vi "Convex Hull 3D (GiftWrap).vi"(0 "Vertices":sgl[][](array[numeric])=[[0.0, 0.0, 0.0], [1.0, 0.0, 0.0], [1.0, 1.0, 0.0], [0.0, 1.0, 0.0], [0.0, 0.0, 1.0], [1.0, 0.0, 1.0], [1.0, 1.0, 1.0], [0.0, 1.0, 1.0], [10.0, 10.0, 0.0], [11.0, 10.0, 0.0], [11.0, 11.0, 0.0], [10.0, 11.0, 0.0], [10.0, 10.0, 1.0], [11.0, 10.0, 1.0], [11.0, 11.0, 1.0], [10.0, 11.0, 1.0]]) -> (1 "Convex hull triangles (partial proc.)":T1[](array[typedef]), 2 "Stack error":errorcluster)   [LabVIEW 2014]
uses:
  Typedefs/Triangle.ctl
  Typedefs/Edge.ctl
  Subroutines/Cross product 3D.vi
  Subroutines/Unit vector.vi
panel:
  # "PN 21/03/2015"
  # "Vertices"
  # "Edges"
  # "Unit normal"
  # "Edge unit normals"
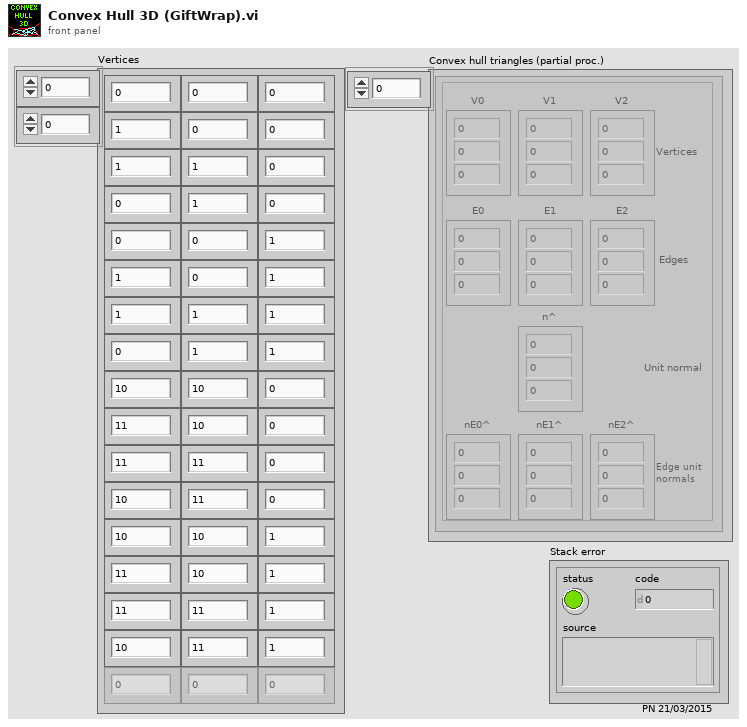
[diagram p1: front panel]
types:
  T1 = typedef "Triangle.ctl" = cluster{"V0":sgl[], "V1":sgl[], "V2":sgl[], "E0":sgl[], "E1":sgl[], "E2":sgl[], "n^":sgl[], "nE0^":sgl[], "nE1^":sgl[], "nE2^":sgl[]}
  T2 = typedef "Edge.ctl" = cluster{"V0":sgl[], "V1":sgl[], "E01":sgl[]}
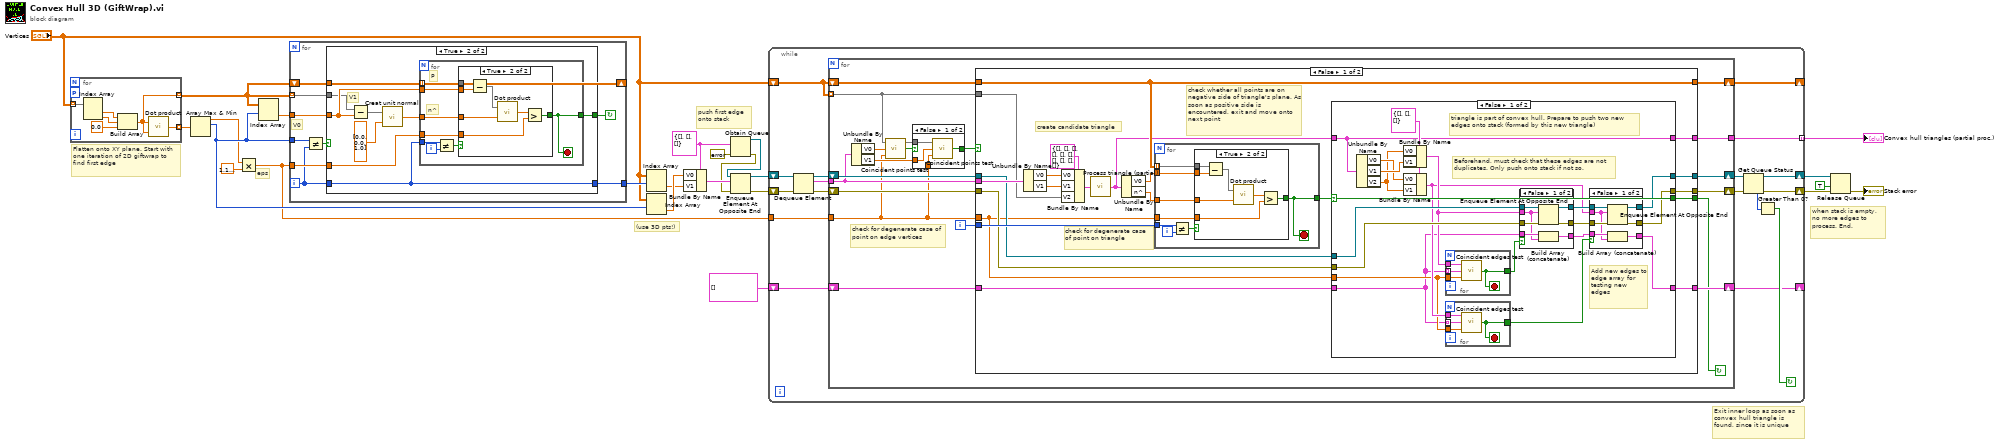
[diagram p0: block diagram]
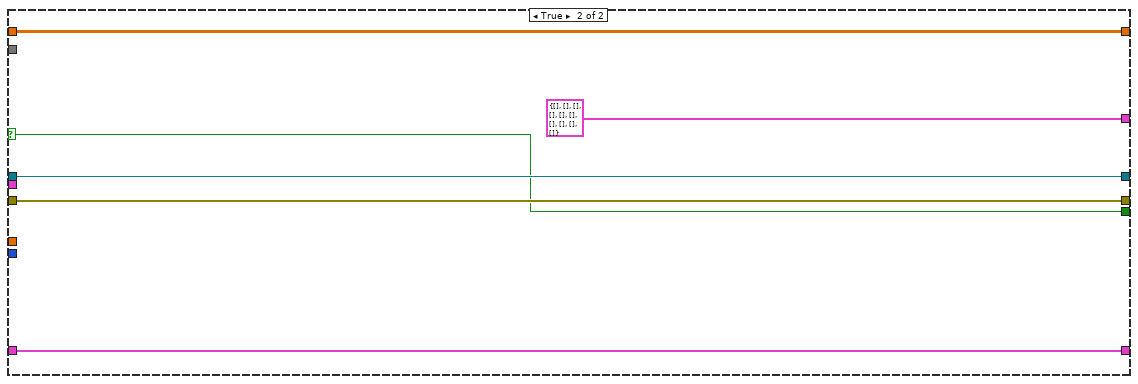
[diagram p7: hidden frame]
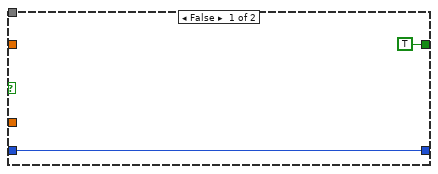
[diagram p8: hidden frame]
diagram:
  w12 = T2 {"V0"=[], "V1"=[], "E01"=[]} ("Edge")
  # "when stack is empty, no more edges to process. End."
  # "Exit inner loop as soon as convex hull triangle is found, since it is unique"
  # "(use 3D pts!)"
  # "push first edge onto stack"
  # "eps"
  # "Flatten onto XY plane. Start with one iteration of 2D giftwrap to find first edge"
  n1 = for {
    tunnel: "Vertices" -> [w30] mode=indexing
    tunnel: [w29] -> w24 mode=indexing
    workers-P: _ -> [_]
    tunnel: [w26] -> w22 mode=indexing
    n2 = Index Array(array=w30) -> (element #1=w28:sgl, element #2=w27:sgl)  [unwired: 2 in]
    n3 = Build Array(w28, w27, sgl 0.0 ("element")) -> (w26:sgl[])
    n4 = call "Dot product.vi"("B"=w26, "A"=w26) -> ("A . B"=w29:sgl)
  }
  n5 = Array Max & Min(array=w24) -> (max value=w4:sgl, max index (indices)=w13:i32)  [unwired: 2 out]
  n6 = Multiply(x=w4, y=sgl 1.1920929e-07) -> (x*y=w5:sgl)
  n7 = Index Array(array=w22, index (row)=w13) -> (element=w23:sgl[])  [unwired: 1 in]
  n8 = for {
    tunnel: w23 -> [w39]
    tunnel: w22 -> [w36] mode=indexing
    shift-right: [w37] -> _
    shift-left: w22 -> [w37]
    tunnel: w5 -> [w38]
    tunnel: [w33] -> w21
    tunnel: w13 -> [w31]
    i -> [w32]
    stop <- w35 continue-if-true
    # "V0"
    n9 = Not Equal?(x=w31, y=w32) -> (x != y?=w34:bool)
    n10 = case shown="True" w34 {
      tunnel: w39 -> [_ w48]
      tunnel: w38 -> [_ w47]
      tunnel: w37 -> [_ w46]
      tunnel: w36 -> [_ w45]
      tunnel: [TRUE w44] -> w35
      tunnel: w32 -> [w40 w42]
      tunnel: [w40 w42] -> w33
      frame False {
      }
      frame True {
        # "V1"
        n11 = Subtract(x=w45, y=w48) -> (x-y=w43:sgl[])
        n12 = call "Creat unit normal.vi"("E2"=sgl[] [0.0, 0.0, 1.0], "E1"=w43) -> ("n^ = (E1 x E2) / ||E1 x E2||"=w49:sgl[])
        n13 = for {
          tunnel: w49 -> [w55]
          tunnel: w46 -> [w54] mode=indexing
          tunnel: w42 -> [w57]
          tunnel: w48 -> [w53]
          tunnel: w47 -> [w52]
          tunnel: [w51] -> w44
          i -> [w58]
          stop <- w51 stop-if-true
          # "n^"
          # "P"
          n14 = Not Equal?(x=w57, y=w58) -> (x != y?=w56:bool)
          n15 = case shown="True" w56 {
            selector: w56 -> [w59 _]
            tunnel: w55 -> [_ w65]
            tunnel: w54 -> [_ w64]
            tunnel: w53 -> [_ w63]
            tunnel: w52 -> [_ w61]
            tunnel: [w59 w60] -> w51
            frame False {
            }
            frame True {
              n16 = Subtract(x=w64, y=w63) -> (x-y=w66:sgl[])
              n17 = call "Dot product.vi"("B"=w65, "A"=w66) -> ("A . B"=w62:sgl)
              n18 = Greater?(x=w62, y=w61) -> (0:w60:bool)
            }
          }
        }
      }
    }
  }
  n19 = Index Array(array="Vertices", index (row)=w21) -> (element=w10:sgl[])  [unwired: 1 in]
  n20 = Index Array(array="Vertices", index (row)=w13) -> (element=w11:sgl[])  [unwired: 1 in]
  n21 = Bundle By Name(cluster=w12, "V0"=w11, "V1"=w10) -> (w18:T2)
  n22 = Obtain Queue(element data type=w12, error in (no error)=errorcluster {"status"=FALSE, "code"=0, "source"=""}) -> (queue out=w19:refnum<queue>, error out=w16:errorcluster)  [unwired: 3 in, 1 out]
  n23 = Enqueue Element At Opposite End(queue=w19, element=w18, error in (no error)=w16) -> (queue out=w8:refnum<queue>, error out=w9:errorcluster)  [unwired: 1 in, 1 out]
  n24 = while {
    shift-right: [w78] -> _
    shift-left: "Vertices" -> [w80]
    shift-right: [w74] -> w15
    shift-left: w8 -> [w83]
    shift-right: [w72] -> w14
    shift-left: w9 -> [w82]
    tunnel: w5 -> [w79]
    tunnel: [w69] -> w3 mode=indexing
    shift-right: [w67] -> _
    shift-left: T2[] [] -> [w68]
    stop <- w70 continue-if-true
    n25 = Dequeue Element(queue=w83, error in (no error)=w82) -> (queue out=w77:refnum<queue>, element=w81:T2, error out=w76:errorcluster)  [unwired: 1 in, 1 out]
    n26 = for {
      tunnel: w80 -> [w89] mode=indexing
      tunnel: w81 -> [w93]
      shift-right: [w99] -> w78
      shift-left: w80 -> [w101]
      tunnel: w79 -> [w87]
      shift-right: [w95] -> w75
      shift-left: w77 -> [w97]
      shift-right: [w94] -> w73
      shift-left: w76 -> [w96]
      tunnel: [w98] -> w69
      shift-right: [w85] -> w67
      shift-left: w68 -> [w86]
      i -> [w100]
      stop <- w84 continue-if-true
      # "check for degenerate case of point on edge vertices"
      n27 = Unbundle By Name(w93) -> ("V0"=w92:sgl[], "V1"=w88:sgl[])
      n28 = call "Coincident points test.vi"("epsilon"=w87, "Point 2"=w92, "Point 1"=w89) -> ("Points are coincident"=w91:bool)
      n29 = case shown="False" w91 {
        selector: w91 -> [_ w106]
        tunnel: [w103 w106] -> w90
        tunnel: w89 -> [w105 _]
        tunnel: w88 -> [w104 _]
        tunnel: w87 -> [w102 _]
        frame False {
          n30 = call "Coincident points test.vi"("epsilon"=w102, "Point 2"=w104, "Point 1"=w105) -> ("Points are coincident"=w103:bool)
        }
        frame True {
        }
      }
      n31 = case shown="False" w90 {
        selector: w90 -> [_ w199]
        tunnel: w93 -> [w116 _]
        tunnel: w89 -> [w107 _]
        tunnel: w101 -> [w121 w202]
        tunnel: w87 -> [w109 _]
        tunnel: w100 -> [w118 _]
        tunnel: [w121 w202] -> w99
        tunnel: [w119 w199] -> w84
        tunnel: [w111 T1 {"V0"=[], "V1"=[], "V2"=[], "E0"=[], "E1"=[], "E2"=[], "n^"=[], "nE0^"=[], "nE1^"=[], "nE2^"=[]} ("Triangle out")] -> w98
        tunnel: w97 -> [w115 w201]
        tunnel: w96 -> [w117 w200]
        tunnel: [w114 w201] -> w95
        tunnel: [w113 w200] -> w94
        tunnel: w86 -> [w110 w198]
        tunnel: [w108 w198] -> w85
        frame False {
          # "check for degenerate case of point on triangle"
          # "check whether all points are on negative side of triangle's plane. As soon as positive side is encountered, exit and move onto next point"
          # "create candidate triangle"
          n32 = Unbundle By Name(w116) -> ("V0"=w126:sgl[], "V1"=w125:sgl[])
          n33 = Bundle By Name(cluster=T1 {"V0"=[], "V1"=[], "V2"=[], "E0"=[], "E1"=[], "E2"=[], "n^"=[], "nE0^"=[], "nE1^"=[], "nE2^"=[]} ("Triangle"), "V0"=w126, "V1"=w125, "V2"=w107) -> (w124:T1)
          n34 = call "Process triangle (partial).vi"("Triangle in"=w124) -> ("Triangle out"=w112:T1)
          n35 = Unbundle By Name(w112) -> ("V0"=w122:sgl[], "n^"=w123:sgl[])
          n36 = for {
            tunnel: w123 -> [w185]
            tunnel: w121 -> [w184] mode=indexing
            tunnel: w118 -> [w187]
            tunnel: w122 -> [w183]
            tunnel: w109 -> [w182]
            tunnel: [w181] -> w120
            i -> [w188]
            stop <- w181 stop-if-true
            n37 = Not Equal?(x=w187, y=w188) -> (x != y?=w186:bool)
            n38 = case shown="True" w186 {
              selector: w186 -> [w189 _]
              tunnel: w185 -> [_ w195]
              tunnel: w184 -> [_ w194]
              tunnel: w183 -> [_ w193]
              tunnel: w182 -> [_ w191]
              tunnel: [w189 w190] -> w181
              frame False {
              }
              frame True {
                n39 = Subtract(x=w194, y=w193) -> (x-y=w196:sgl[])
                n40 = call "Dot product.vi"("B"=w195, "A"=w196) -> ("A . B"=w192:sgl)
                n41 = Greater?(x=w192, y=w191) -> (0:w190:bool)
              }
            }
          }
          n42 = case shown="False" w120 {
            selector: w120 -> [w147 w180]
            tunnel: [w147 w180] -> w119
            tunnel: w117 -> [w142 w178]
            tunnel: w115 -> [w144 w179]
            tunnel: [w143 w179] -> w114
            tunnel: [w141 w178] -> w113
            tunnel: w112 -> [w136 w177]
            tunnel: [w136 w177] -> w111
            tunnel: w110 -> [w131 w176]
            tunnel: w109 -> [w133 _]
            tunnel: [w129 w176] -> w108
            frame False {
              w140 = T2 {"V0"=[], "V1"=[], "E01"=[]} ("Edge")
              # "Add new edges to edge array for testing new edges"
              # "Beforehand, must check that these edges are not duplicates. Only push onto stack if not so."
              # "triangle is part of convex hull. Prepare to push two new edges onto stack (formed by this new triangle)"
              n43 = Unbundle By Name(w136) -> ("V0"=w138:sgl[], "V1"=w139:sgl[], "V2"=w137:sgl[])
              n44 = Bundle By Name(cluster=w140, "V0"=w137, "V1"=w139) -> (w135:T2)
              n45 = Bundle By Name(cluster=w140, "V0"=w138, "V1"=w137) -> (w134:T2)
              n46 = for {
                tunnel: w131 -> [w175] mode=indexing
                tunnel: w135 -> [w174]
                tunnel: w133 -> [w173]
                tunnel: [w172] -> w132
                stop <- w172 stop-if-true
                n47 = call "Coincident edges test.vi"("epsilon"=w173, "Edge 2"=w175, "Edge 1"=w174) -> ("Edges are coincident"=w172:bool)
              }
              n48 = for {
                tunnel: w131 -> [w171] mode=indexing
                tunnel: w134 -> [w170]
                tunnel: w133 -> [w169]
                tunnel: [w168] -> w128
                stop <- w168 stop-if-true
                n49 = call "Coincident edges test.vi"("epsilon"=w169, "Edge 2"=w171, "Edge 1"=w170) -> ("Edges are coincident"=w168:bool)
              }
              n50 = case shown="False" w132 {
                tunnel: [w164 w167] -> w146
                tunnel: [w163 w166] -> w145
                tunnel: w144 -> [w162 w167]
                tunnel: w142 -> [w161 w166]
                tunnel: w135 -> [w159 _]
                tunnel: w131 -> [w160 w165]
                tunnel: [w158 w165] -> w130
                frame False {
                  n51 = Enqueue Element At Opposite End(queue=w162, element=w159, error in (no error)=w161) -> (queue out=w164:refnum<queue>, error out=w163:errorcluster)  [unwired: 1 in, 1 out]
                  n52 = Build Array (concatenate)(w160, w159) -> (w158:T2[])
                }
                frame True {
                }
              }
              n53 = case shown="False" w128 {
                tunnel: w146 -> [w154 w157]
                tunnel: w145 -> [w153 w156]
                tunnel: [w152 w157] -> w143
                tunnel: [w151 w156] -> w141
                tunnel: w134 -> [w149 _]
                tunnel: w130 -> [w150 w155]
                tunnel: [w148 w155] -> w129
                frame False {
                  n54 = Enqueue Element At Opposite End(queue=w154, element=w149, error in (no error)=w153) -> (queue out=w152:refnum<queue>, error out=w151:errorcluster)  [unwired: 1 in, 1 out]
                  n55 = Build Array (concatenate)(w150, w149) -> (w148:T2[])
                }
                frame True {
                }
              }
            }
            frame True {
              # "Triangle does not form the convex hull, do nothing and just move on to next point"
            }
          }
        }
        frame True {
        }
      }
    }
    n56 = Get Queue Status(queue=w75, error in (no error)=w73) -> (queue out=w74:refnum<queue>, error out=w72:errorcluster, # elements in queue=w71:i32)  [unwired: 1 in, 5 out]
    n57 = Greater Than 0?(x=w71) -> (x > 0?=w70:bool)
  }
  "Convex hull triangles (partial proc.)" <- w3
  n58 = Release Queue(queue=w15, force destroy? (F)=TRUE, error in (no error)=w14) -> (error out=→"Stack error":errorcluster)  [unwired: 2 out]
